vi "DriveMotors.vi"(6 "Profile":u8=128 format="%.0x", 8 "error in (no error)":errorcluster, 9 "LeftSpeed":dbl, 10 "RightSpeed":dbl, 11 "RobotDriveDevRef 2":T1={"DevStatus"={"status"=FALSE, "code"=0, "source"=""}, "Motors[]"=[], "Square Inputs"=FALSE, "Max Output"=1.0}) -> (0 "error out":errorcluster, 2 "Motor Values":dbl[](array[numeric]), 3 "RobotDriveDevRef":T1={"DevStatus"={"status"=FALSE, "code"=0, "source"=""}, "Motors[]"=[], "Square Inputs"=FALSE, "Max Output"=1.0})   [LabVIEW 2015]
uses:
  <vilib>/Rock Robotics/WPI/RobotDrive/WPI_RobotDriveDevRef.ctl
  <vilib>/Rock Robotics/WPI/MotorControl/WPI_MotorControlDeviceRef.ctl
  <vilib>/Rock Robotics/WPI/MotorControl/WPI_MotorControlType.ctl
  <vilib>/Rock Robotics/SystemInterfaces/DIO/FPGA_DIOPWMChannel.ctl
  <vilib>/Rock Robotics/WPI/PWM/WPI_PWMDeadband.ctl
  <vilib>/Rock Robotics/WPI/CAN/Jaguar/SubVIs/WPI_CANJaguar_ControlMode.ctl
  <vilib>/Rock Robotics/WPI/CAN/TalonSRX/WPI_CANTalonSRX_APIControlMode.ctl
  <vilib>/Rock Robotics/WPI/RobotDrive/WPI_RobotDriveMotorSelectorEnum.ctl
  <vilib>/Rock Robotics/WPI/RobotDrive/WPI_RobotDriveSafetyCheck.vi
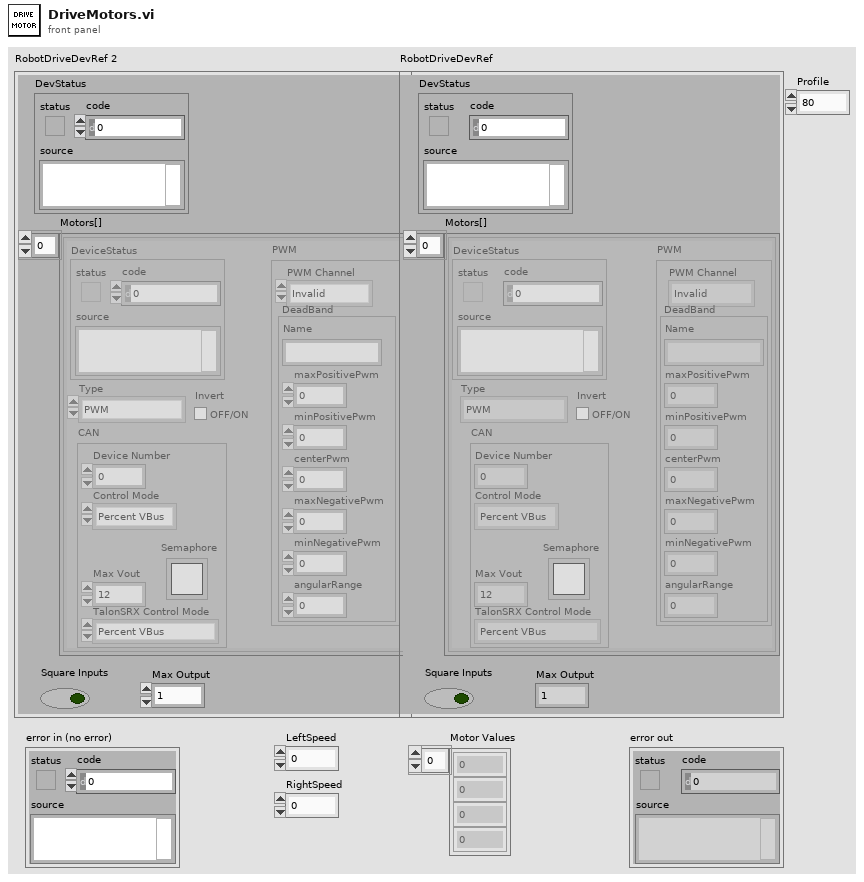
[diagram p1: front panel]
types:
  T1 = typedef "WPI_RobotDriveDevRef.ctl" = cluster{"DevStatus":errorcluster, "Motors[]":T2[], "Square Inputs":bool, "Max Output":dbl}
  T2 = typedef "WPI_MotorControlDeviceRef.ctl" = cluster{"DeviceStatus":errorcluster, "Type":T3, "PWM":cluster{"PWM Channel":T4, "DeadBand":T5}, "CAN":cluster{"Device Number":u8, "Control Mode":T6, "Semaphore":T7, "Max Vout":dbl, "TalonSRX Control Mode":T8}, "Invert":bool}
  T3 = typedef "WPI_MotorControlType.ctl" = enum16{"PWM", "CAN", "CANTalonSRX"}
  T4 = typedef "FPGA_DIOPWMChannel.ctl" = enum8{"PWM 0", "PWM 1", "PWM 2", "PWM 3", "PWM 4", "PWM 5", "PWM 6", "PWM 7", "PWM 8", "PWM 9", "PWM MXP 0", "PWM MXP 1", "PWM MXP 2", "PWM MXP 3", "PWM MXP 4", "PWM MXP 5", "PWM MXP 6", "PWM MXP 7", "PWM MXP 8", "PWM MXP 9", "Invalid"}
  T5 = typedef "WPI_PWMDeadband.ctl" = cluster{"Name":string, "maxPositivePwm":i32, "minPositivePwm":i32, "centerPwm":i32, "maxNegativePwm":i32, "minNegativePwm":i32, "angularRange":u16}
  T6 = typedef "WPI_CANJaguar_ControlMode.ctl" = enum8{"Percent VBus", "Current", "Speed", "Position", "Voltage"}
  T7 = typedef "Semaphore RefNum" = refnum<k1>
  T8 = typedef "WPI_CANTalonSRX_APIControlMode.ctl" = enum8{"Percent VBus", "Speed", "Position", "Slave", "Unchanged / Invalid", "Voltage Compensation", "Current", "Motion Profile"}
  T9 = typedef "WPI_RobotDriveMotorSelectorEnum.ctl" = enum16{"Rear Left Motor", "Rear Right Motor", "Front Left Motor", "Front Right Motor"}
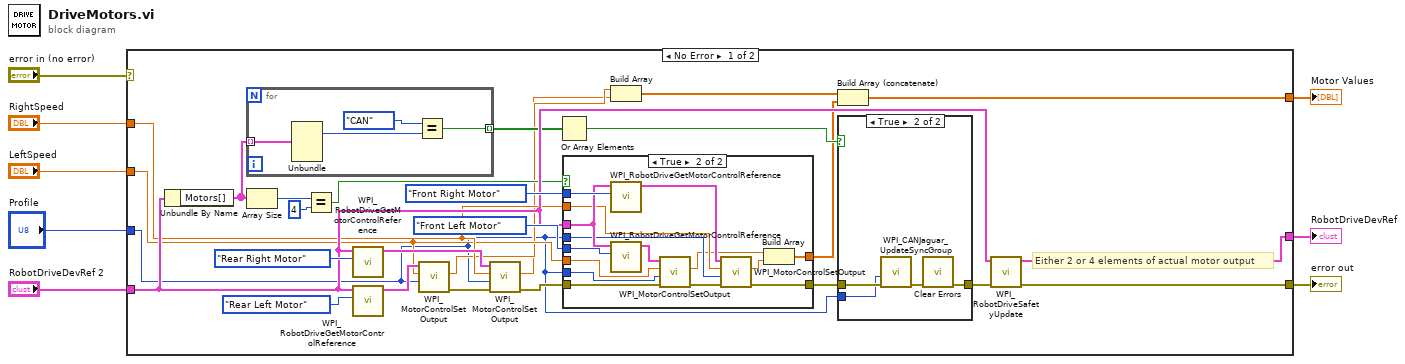
[diagram p0: block diagram]
diagram:
  n1 = case shown="No Error" "error in (no error)" {
    selector: "error in (no error)" -> [_ w62]
    tunnel: "RobotDriveDevRef 2" -> [w27 w61]
    tunnel: [w10 w61] -> w7
    tunnel: "LeftSpeed" -> [w25 _]
    tunnel: "RightSpeed" -> [w26 _]
    tunnel: [w11 w62] -> w3
    tunnel: [w13 _] -> w2
    tunnel: "Profile" -> [w9 _]
    frame No Error {
      # "Either 2 or 4 elements of actual motor output"
      n2 = Unbundle By Name(w27) -> ("Motors[]"=w23:T2[])
      n3 = for {
        tunnel: w23 -> [w39] mode=indexing
        tunnel: [w36] -> w22 mode=indexing
        n4 = Unbundle(w39) -> ("Type"=w38:T3)  [unwired: 4 out]
        n5 = Equal?(x=enum16{"PWM", "CAN"}."CAN" ("Type"), y=w38) -> (x = y?=w36:bool)
      }
      n6 = Array Size(array=w23) -> (size(s)=w35:i32)
      n7 = Equal?(x=w35, y=4) -> (x = y?=w24:bool)
      n8 = call <vilib>:"WPI_RobotDriveGetMotorControlReference.vi"("MotorIndex"=WPI_RobotDriveMotorSelectorEnum."Rear Right Motor", "RobotDriveDevRef"=w27) -> ("MotorControlDeviceRef"=w33:T2)  [unwired: 9 out]
      n9 = call <vilib>:"WPI_RobotDriveGetMotorControlReference.vi"("MotorIndex"=WPI_RobotDriveMotorSelectorEnum."Rear Left Motor", "RobotDriveDevRef"=w27) -> ("MotorControlDeviceRef"=w32:T2)  [unwired: 9 out]
      n10 = call <vilib>:"WPI_MotorControlSetOutput.vi"("Sync Group / Parameter Slot"=w9, "Output"=w25, "MotorControlDevRef"=w32) -> ("error out"=w20:errorcluster, "Motor Output"=w17:dbl)  [unwired: 2 in, 5 out]
      n11 = call <vilib>:"WPI_MotorControlSetOutput.vi"("error in (no error)"=w20, "Sync Group / Parameter Slot"=w9, "Output"=w26, "MotorControlDevRef"=w33) -> ("error out"=w18:errorcluster, "Motor Output"=w16:dbl)  [unwired: 1 in, 5 out]
      n12 = Or Array Elements(Boolean array=w22) -> (logical OR=w21:bool)
      n13 = case shown="True" w24 {
        tunnel: WPI_RobotDriveMotorSelectorEnum."Front Left Motor" ("MotorIndex") -> [_ w60]
        tunnel: WPI_RobotDriveMotorSelectorEnum."Front Right Motor" ("MotorIndex") -> [_ w59]
        tunnel: w27 -> [_ w58]
        tunnel: w9 -> [_ w57]
        tunnel: w26 -> [_ w56]
        tunnel: w25 -> [_ w55]
        tunnel: [w45 w51] -> w19
        tunnel: w9 -> [_ w52]
        tunnel: w18 -> [w45 w49]
        tunnel: [_ w46] -> w15
        frame False {
        }
        frame True {
          n14 = call <vilib>:"WPI_RobotDriveGetMotorControlReference.vi"("MotorIndex"=w59, "RobotDriveDevRef"=w58) -> ("MotorControlDeviceRef"=w54:T2)  [unwired: 9 out]
          n15 = call <vilib>:"WPI_RobotDriveGetMotorControlReference.vi"("MotorIndex"=w60, "RobotDriveDevRef"=w58) -> ("MotorControlDeviceRef"=w53:T2)  [unwired: 9 out]
          n16 = call <vilib>:"WPI_MotorControlSetOutput.vi"("error in (no error)"=w49, "Sync Group / Parameter Slot"=w52, "Output"=w55, "MotorControlDevRef"=w53) -> ("error out"=w50:errorcluster, "Motor Output"=w47:dbl)  [unwired: 1 in, 5 out]
          n17 = call <vilib>:"WPI_MotorControlSetOutput.vi"("error in (no error)"=w50, "Sync Group / Parameter Slot"=w57, "Output"=w56, "MotorControlDevRef"=w54) -> ("error out"=w51:errorcluster, "Motor Output"=w48:dbl)  [unwired: 1 in, 5 out]
          n18 = Build Array(w47, w48) -> (w46:dbl[])
        }
      }
      n19 = Build Array(w17, w16) -> (w14:dbl[])
      n20 = Build Array (concatenate)(w14, w15) -> (w13:dbl[])
      n21 = case shown="True" w21 {
        tunnel: w19 -> [w40 w43]
        tunnel: w9 -> [_ w42]
        tunnel: [w40 w41] -> w12
        frame False {
        }
        frame True {
          n22 = call <vilib>:"WPI_CANJaguar_UpdateSyncGroup.vi"("error in (no error)"=w43, "Sync Group"=w42) -> ("error out"=w44:errorcluster)  [unwired: 9 out]
          n23 = call <vilib>:"Clear Errors.vi"("error in (no error)"=w44) -> ("error out"=w41:errorcluster)  [unwired: 1 in, 5 out]
        }
      }
      n24 = call <vilib>:"WPI_RobotDriveSafetyUpdate.vi"("error in (no error)"=w12, "RobotDriveDevRef"=w27) -> ("error out"=w11:errorcluster, "RobotDriveDevRef"=w10:T1)  [unwired: 8 out]
    }
    frame Error {
    }
  }
  "RobotDriveDevRef" <- w7
  "error out" <- w3
  "Motor Values" <- w2
